vi "Close.vi"(8 "error in (no error)":errorcluster, 11 "XNET Base CFG in":refnum<class "XNET Base CFG.lvclass">) -> (0 "error out":errorcluster, 3 "XNET Base CFG out":refnum<class "XNET Base CFG.lvclass">)   [LabVIEW 2023, in "XNET Base CFG.lvclass"]
uses:
  XNET Base CFG.lvclass
  XNET Base CFG.lvclass/XNET Base CFG.ctl
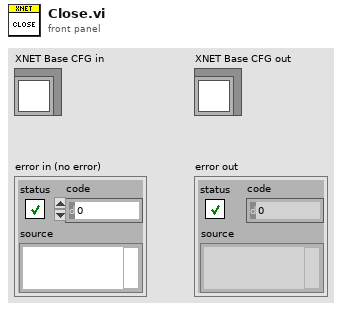
[diagram p1: front panel]
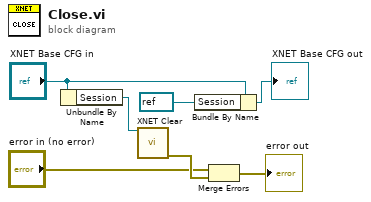
[diagram p0: block diagram]
diagram:
  n1 = Unbundle By Name("XNET Base CFG in") -> ("Session"=w6:refnum<k21>)
  n2 = call <vilib>:"XNET Clear.vi"("session in"=w6) -> ("error out"=w7:errorcluster)  [unwired: 14 in]
  n3 = Bundle By Name(cluster="XNET Base CFG in", "Session"=refnum<k21> refnum ("session")) -> (→"XNET Base CFG out":refnum<class "XNET Base CFG.lvclass">)
  n4 = Merge Errors("error in (no error)", w7) -> (→"error out":errorcluster)
